vi "ReciveThread.vi"() -> ()   [LabVIEW 2011]
uses:
  VIs/_USB_CAN_T_R_Unit_.ctl
  VIs/_USB_CAN_GLOBAL_.vi
  data/ControlCAN.dll
panel:
  in  "RcvLen":i32=48
  in  "Enable2":bool=TRUE
  in  "Enable1":bool=TRUE
  in  "channels":i32=2
  in  "Scan time":u32=30
  in  "RFun":u16
  in  "DeviceInd":u32
  in  "type":u16(ring)=2 items=["USB-CAN"=2, "USB-CAN2.0"=3]
  in  "VCI_CAN_OBJ_R":u8[](array[numeric])=array[5000 elements]
  # "typedef struct _VCI_CAN_OBJ {\nBYTE ID[4];\nUINT TimeStamp;\nBYTE TimeFlag;\nBYTE SendType;\nBYTE RemoteFlag;\nBYTE ExternFlag;\nBYTE DataLen;\nBYTE Data[8];\nBYTE Reserved[3];} VCI_CAN_OBJ, *PVCI_CAN_OBJ;"
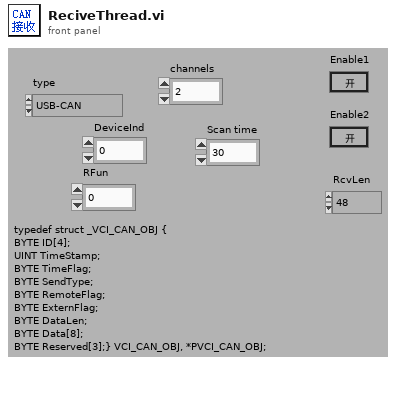
[diagram p1: front panel]
types:
  T1 = enum16{"open", "replace", "create", "open or create", "replace or create", "replace or create with confirmation"}
  T2 = typedef "_USB_CAN_T_R_Unit_.ctl" = cluster{"time":timestamp, "channel":u16, "TimeStamp":u32, "tr":enum16{"接收", "发送"}, "id":u32, "Type":enum16{"数据帧", "远程帧"}, "Format":enum16{"标准帧", "扩展帧"}, "len":u8, "data":u8[]}
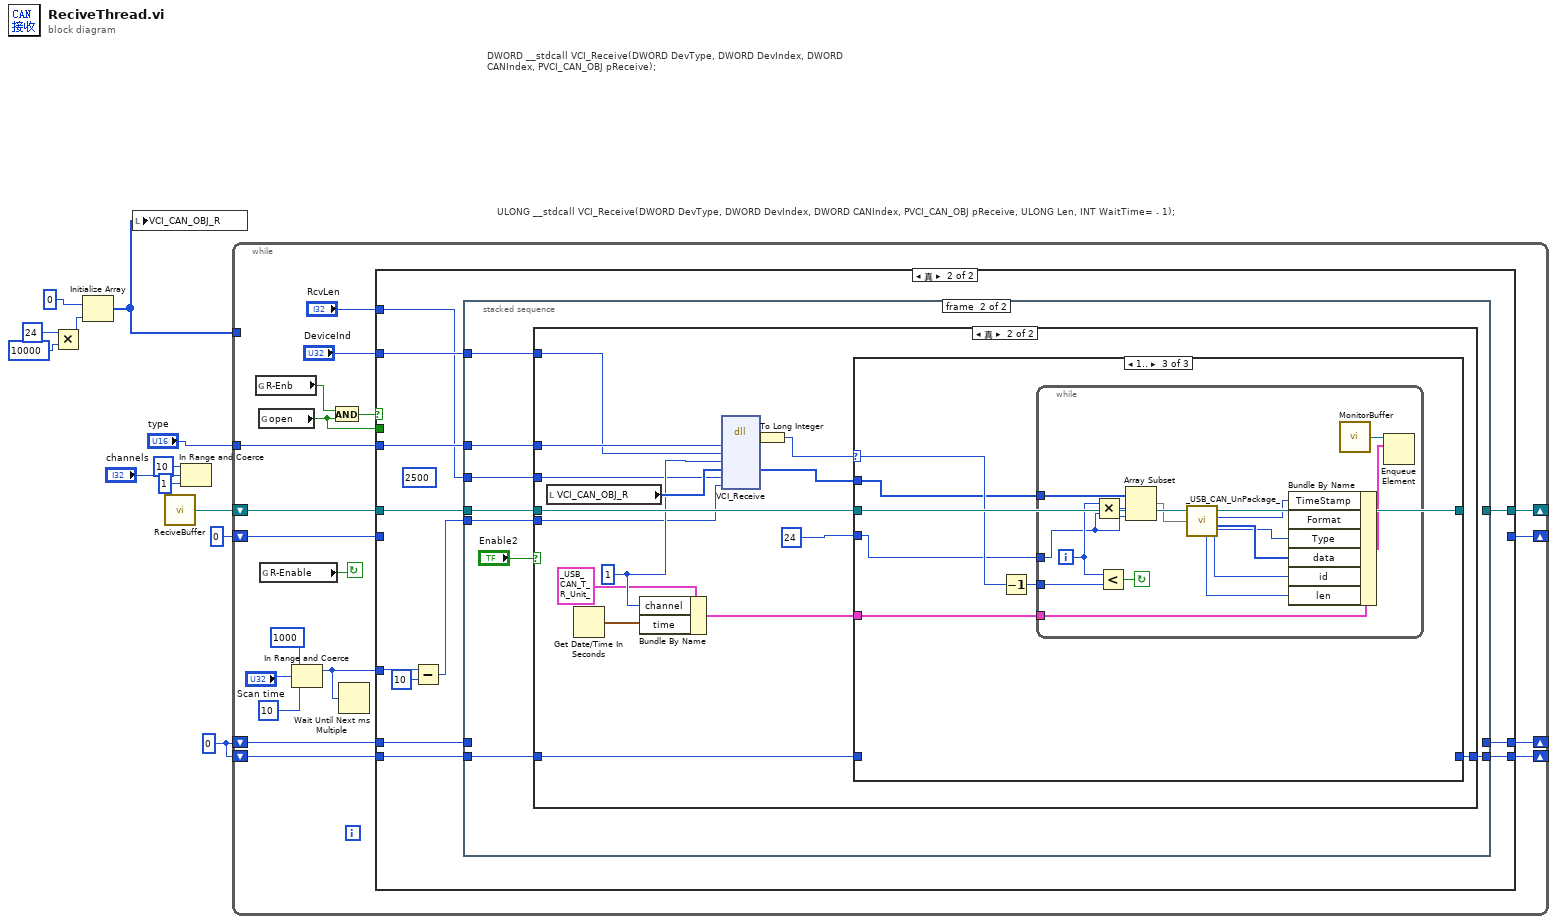
[diagram p0: block diagram]
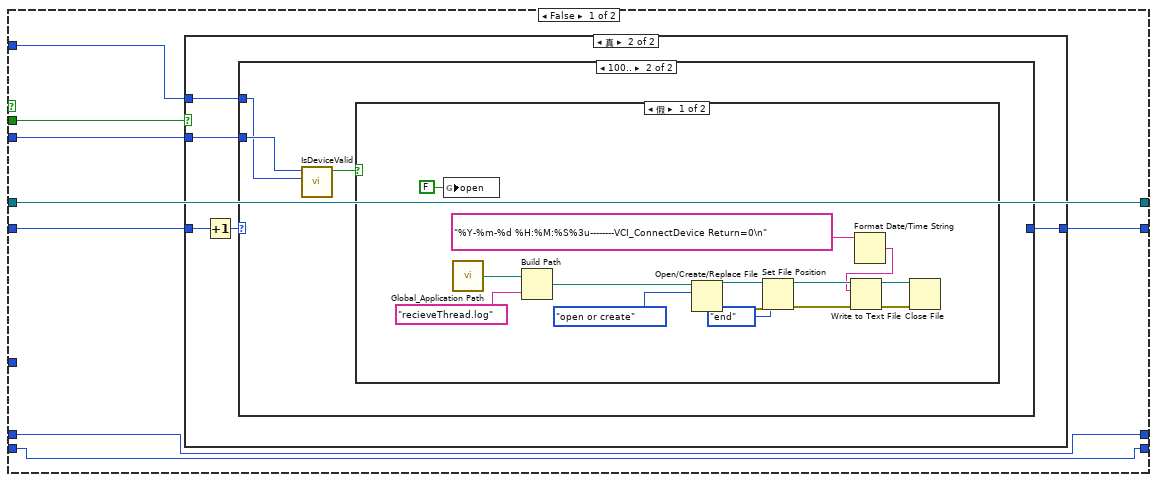
[diagram p2: hidden frame]
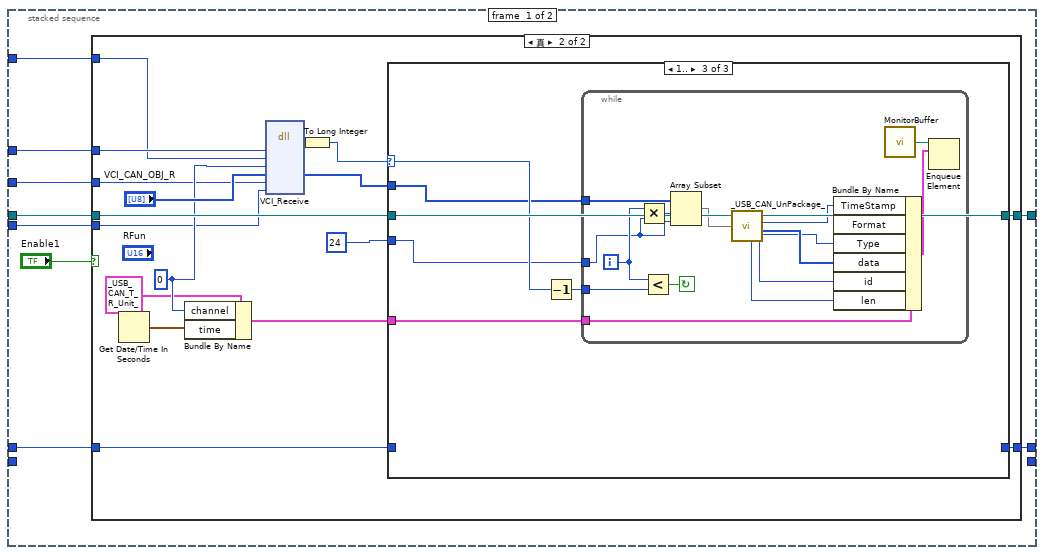
[diagram p6: hidden frame]
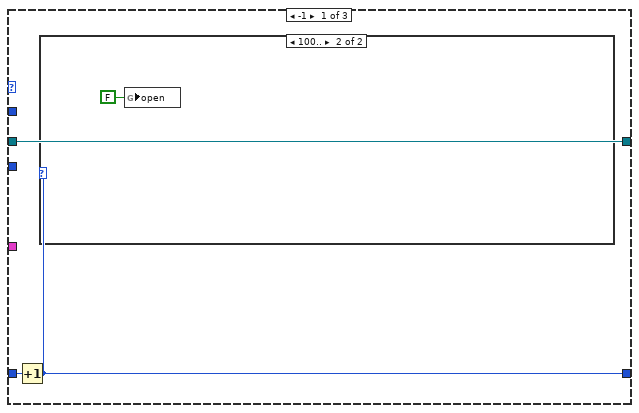
[diagram p8: hidden frame]
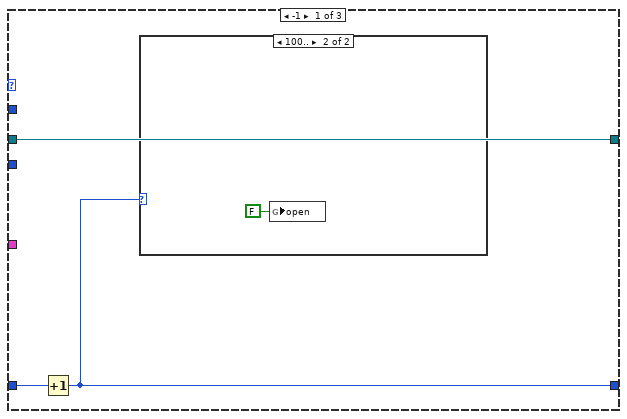
[diagram p12: hidden frame]
diagram:
  w1 = 0
  # "ULONG __stdcall VCI_Receive(DWORD DevType, DWORD DevIndex, DWORD CANIndex, PVCI_CAN_OBJ pReceive, ULONG Len, INT WaitTime=－1);"
  # "DWORD __stdcall VCI_Receive(DWORD DevType, DWORD DevIndex, DWORD\nCANIndex, PVCI_CAN_OBJ pReceive);"
  n1 = Multiply(x=24, y=10000 ("维数大小")) -> (x*y=w10:i32)
  n2 = Initialize Array(u8 0, w10) -> (w11:u8[])
  n3 = local write "VCI_CAN_OBJ_R"(w11) -> ()
  n4 = call "ReciveBuffer.vi"() -> ("VCI_USB_CAN_T_BUF_R"=w7:refnum<queue>)  [unwired: 1 in]
  n5 = In Range and Coerce(upper limit=10 ("上限"), x="channels", lower limit=1 ("下限")) -> ()  [unwired: 2 out]
  n6 = while {
    shift-right: [w30] -> _
    shift-left: w7 -> [w31]
    tunnel: "type" -> [w29]
    tunnel: w11 -> [_]
    shift-right: [w24] -> _
    shift-left: 0 -> [w25]
    shift-right: [w17] -> _
    shift-left: w1 -> [w18]
    shift-right: [w15] -> _
    shift-left: w1 -> [w16]
    stop <- w19 continue-if-true
    n7 = global read "_USB_CAN_GLOBAL_.vi" "R-Enb"() -> (w27:bool)
    n8 = global read "_USB_CAN_GLOBAL_.vi" "open"() -> (w26:bool)
    n9 = global read "_USB_CAN_GLOBAL_.vi" "R-Enable"() -> (w19:bool)
    n10 = In Range and Coerce(upper limit=u32 1000 ("上限"), x="Scan time", lower limit=u32 10 ("下限")) -> (coerced(x)=w13:u32)  [unwired: 1 out]
    n11 = And(x=w27, y=w26) -> (x .and. y?=w28:bool)
    n12 = Wait Until Next ms Multiple(millisecond multiple=w13) -> ()  [unwired: 1 out]
    n13 = case shown="真" w28 {
      tunnel: w29 -> [w35 w74]
      tunnel: w31 -> [w39 w73]
      tunnel: [w39 w72] -> w30
      tunnel: w26 -> [w38 _]
      tunnel: w25 -> [w37 _]
      tunnel: [w36 _] -> w24
      tunnel: "DeviceInd" -> [w34 w71]
      tunnel: w18 -> [w33 w70]
      tunnel: [w33 w69] -> w17
      tunnel: w16 -> [w32 w68]
      tunnel: [w32 w67] -> w15
      tunnel: w13 -> [_ w66]
      tunnel: "RcvLen" -> [_ w63]
      frame False {
        n14 = case shown="真" w38 {
          tunnel: w37 -> [_ w44]
          tunnel: [_ w42] -> w36
          tunnel: w35 -> [_ w41]
          tunnel: w34 -> [_ w40]
          frame False {
          }
          frame True {
            n15 = Increment(x=w44) -> (x+1=w43:i32)
            n16 = case shown="100.." w43 {
              selector: w43 -> [w45 _]
              tunnel: [w45 _] -> w42
              tunnel: w41 -> [_ w48]
              tunnel: w40 -> [_ w47]
              frame 0, Default {
              }
              frame 100.. {
                n17 = call "IsDeviceValid.vi"("DeviceInd"=w47, "type"=w48) -> ("Valid"=w46:bool)  [unwired: 8 in, 1 out]
                n18 = case shown="假" w46 {
                  frame False {
                    n19 = global write "_USB_CAN_GLOBAL_.vi" "open"(FALSE ("open")) -> ()
                    n20 = call "Global_Application Path.vi"() -> ("程序路径"=w51:path)  [unwired: 1 in]
                    n21 = Build Path(base path=w51, name or relative path="recieveThread.log" ("名称或相对路径")) -> (appended path=w60:path)
                    n22 = Open/Create/Replace File(file path (use dialog)=w60, operation (0:open)=T1."open or create" ("操作(0:open)")) -> (refnum out=w58:refnum<file>, error out=w57:errorcluster)  [unwired: 4 in, 1 out]
                    n23 = Set File Position(refnum=w58, from (0:start)=enum16{"start", "end", "current"}."end" ("自（0:起始）"), error in=w57) -> (refnum out=w55:refnum<file>, error out=w54:errorcluster)  [unwired: 1 in]
                    n24 = Format Date/Time String(time format string (%c)="%Y-%m-%d %H:%M:%S%3u--------VCI_ConnectDevice Return=0\n" ("时间格式字符串(%c)")) -> (date/time string=w49:string)  [unwired: 2 in]
                    n25 = Write to Text File(file (use dialog)=w55, text=w49, error in=w54) -> (refnum out=w52:refnum<file>, error out=w53:errorcluster)  [unwired: 1 in, 1 out]
                    n26 = Close File(refnum=w52, error in=w53) -> ()  [unwired: 2 out]
                  }
                  frame True {
                  }
                }
              }
            }
          }
        }
      }
      frame True {
        (unwired) u32 2500 ("Len")
        n27 = Subtract(x=w66, y=u32 10) -> (x-y=w64:u32)
        n28 = stacked-sequence {
          tunnel: w74 -> [w83 w136]
          tunnel: w73 -> [w82 w135]
          tunnel: [w81 _] -> w72
          tunnel: w71 -> [w80 w134]
          tunnel: w63 -> [w78 w132]
          tunnel: w64 -> [w77 w131]
          tunnel: w70 -> [w76 _]
          tunnel: [w75 _] -> w69
          tunnel: w68 -> [_ w130]
          tunnel: [_ w129] -> w67
          frame #0 {
            n29 = case shown="真" "Enable1" {
              tunnel: w83 -> [_ w101]
              tunnel: w82 -> [w84 w100]
              tunnel: [w84 w99] -> w81
              tunnel: w80 -> [_ w98]
              tunnel: w78 -> [_ w91]
              tunnel: w77 -> [_ w90]
              tunnel: w76 -> [_ w88]
              tunnel: [_ w87] -> w75
              frame False {
              }
              frame True {
                w92 = 0
                n30 = Get Date/Time In Seconds() -> (seconds since 1Jan1904=w94:timestamp)
                n31 = Bundle By Name(cluster=T2 {"time"=timestamp(0 s since 1904-01-01), "channel"=0, "TimeStamp"=0, "tr"=enum."接收", "id"=0, "Type"=enum."数据帧", "Format"=enum."标准帧", "len"=0, "data"=[]} ("TR_Unit"), "channel"=w92, "time"=w94) -> (w93:T2)
                n32 = dll-call lib="PTH1vabs E工作USB-CAN Tool上位机源码USB-CAN Tool工具源码ZLG版USB CAN TooldataControlCAN.dll" fn="VCI_Receive"("DeviceType"=w101, "DeviceInd"=w98, "CANInd"=w92, "pReceive"="VCI_CAN_OBJ_R", "Len"=w91, "WaitTime"=w90) -> ("返回类型"=w85:u32, "pReceive"=w97:u8[])  [unwired: 8 in, 2 out]
                n33 = To Long Integer(number=w85) -> (32bit integer=w86:i32)
                n34 = case shown="1.." w86 {
                  selector: w86 -> [_ _ w111]
                  tunnel: w97 -> [_ _ w110]
                  tunnel: w100 -> [w104 w106 w112]
                  tunnel: [w104 w106 w112] -> w99
                  tunnel: 24 ("y") -> [_ _ w108]
                  tunnel: w93 -> [_ _ w107]
                  tunnel: w88 -> [w103 _ _]
                  tunnel: [w102 _ _] -> w87
                  frame -1 {
                    n35 = Increment(x=w103) -> (x+1=w102:i32)
                    n36 = case shown="100.." w102 {
                      frame 0, Default {
                      }
                      frame 100.. {
                        n37 = global write "_USB_CAN_GLOBAL_.vi" "open"(FALSE ("open")) -> ()
                      }
                    }
                  }
                  frame 0, Default {
                  }
                  frame 1.. {
                    n38 = Decrement(x=w111) -> (x-1=w109:i32)
                    n39 = while {
                      tunnel: w109 -> [w126]
                      tunnel: w110 -> [w125]
                      tunnel: w107 -> [w122]
                      tunnel: w108 -> [w114]
                      i -> [w124]
                      stop <- w127 continue-if-true
                      n40 = Multiply(x=w124, y=w114) -> (x*y=w128:i32)
                      n41 = Less?(x=w124, y=w126) -> (x < y?=w127:bool)
                      n42 = Array Subset(array=w125, index=w128, length=w114) -> (w123:u8[])
                      n43 = call "_USB_CAN_UnPackage_.vi"("source"=w123) -> ("length"=w118:i32, "Type"=w115:enum16{"数据帧", "远程帧"}, "Format"=w116:enum16{"标准帧", "扩展帧"}, "TimeStamp"=w113:u32, "data"=w121:u8[], "ID"=w117:u32)
                      n44 = Bundle By Name(cluster=w122, "TimeStamp"=w113, "Format"=w116, "Type"=w115, "data"=w121, "id"=w117, "len"=w118) -> (w119:T2)
                      n45 = call "MonitorBuffer.vi"() -> ("USB_CAN_M_BUF"=w120:refnum<queue>)  [unwired: 1 in]
                      n46 = Enqueue Element(queue=w120, element=w119) -> ()  [unwired: 2 in, 3 out]
                    }
                  }
                }
              }
            }
          }
          frame #1 {
            n47 = case shown="真" "Enable2" {
              tunnel: w136 -> [_ w152]
              tunnel: w135 -> [_ w151]
              tunnel: w134 -> [_ w150]
              tunnel: w132 -> [_ w143]
              tunnel: w131 -> [_ w142]
              tunnel: w130 -> [_ w140]
              tunnel: [_ w139] -> w129
              frame False {
              }
              frame True {
                w144 = 1
                n48 = local read "VCI_CAN_OBJ_R"() -> (w145:u8[])
                n49 = Get Date/Time In Seconds() -> (seconds since 1Jan1904=w147:timestamp)
                n50 = Bundle By Name(cluster=T2 {"time"=timestamp(0 s since 1904-01-01), "channel"=0, "TimeStamp"=0, "tr"=enum."接收", "id"=0, "Type"=enum."数据帧", "Format"=enum."标准帧", "len"=0, "data"=[]} ("TR_Unit"), "channel"=w144, "time"=w147) -> (w146:T2)
                n51 = dll-call lib="PTH1vabs E工作USB-CAN Tool上位机源码USB-CAN Tool工具源码ZLG版USB CAN TooldataControlCAN.dll" fn="VCI_Receive"("DeviceType"=w152, "DeviceInd"=w150, "CANInd"=w144, "pReceive"=w145, "Len"=w143, "WaitTime"=w142) -> ("返回类型"=w137:u32, "pReceive"=w149:u8[])  [unwired: 8 in, 2 out]
                n52 = To Long Integer(number=w137) -> (32bit integer=w138:i32)
                n53 = case shown="1.." w138 {
                  selector: w138 -> [_ _ w162]
                  tunnel: w149 -> [_ _ w161]
                  tunnel: w151 -> [w155 w157 w163]
                  tunnel: [w155 w157 w163] -> _
                  tunnel: 24 ("y") -> [_ _ w159]
                  tunnel: w146 -> [_ _ w158]
                  tunnel: w140 -> [w154 _ _]
                  tunnel: [w153 _ _] -> w139
                  frame -1 {
                    n54 = Increment(x=w154) -> (x+1=w153:i32)
                    n55 = case shown="100.." w153 {
                      frame 0, Default {
                      }
                      frame 100.. {
                        n56 = global write "_USB_CAN_GLOBAL_.vi" "open"(FALSE ("open")) -> ()
                      }
                    }
                  }
                  frame 0, Default {
                  }
                  frame 1.. {
                    n57 = Decrement(x=w162) -> (x-1=w160:i32)
                    n58 = while {
                      tunnel: w160 -> [w177]
                      tunnel: w161 -> [w176]
                      tunnel: w158 -> [w173]
                      tunnel: w159 -> [w165]
                      i -> [w175]
                      stop <- w178 continue-if-true
                      n59 = Multiply(x=w175, y=w165) -> (x*y=w179:i32)
                      n60 = Less?(x=w175, y=w177) -> (x < y?=w178:bool)
                      n61 = Array Subset(array=w176, index=w179, length=w165) -> (w174:u8[])
                      n62 = call "_USB_CAN_UnPackage_.vi"("source"=w174) -> ("length"=w169:i32, "Type"=w166:enum16{"数据帧", "远程帧"}, "Format"=w167:enum16{"标准帧", "扩展帧"}, "TimeStamp"=w164:u32, "data"=w172:u8[], "ID"=w168:u32)
                      n63 = Bundle By Name(cluster=w173, "TimeStamp"=w164, "Format"=w167, "Type"=w166, "data"=w172, "id"=w168, "len"=w169) -> (w170:T2)
                      n64 = call "MonitorBuffer.vi"() -> ("USB_CAN_M_BUF"=w171:refnum<queue>)  [unwired: 1 in]
                      n65 = Enqueue Element(queue=w171, element=w170) -> ()  [unwired: 2 in, 3 out]
                    }
                  }
                }
              }
            }
          }
        }
      }
    }
  }
